vi "FetchMultiPoint.vi"(8 "error in (no error)":errorcluster, 11 "NISTSimulation in":refnum<class "Simulation.lvclass">) -> (0 "error out":errorcluster, 3 "NISTSimulation out":refnum<class "Simulation.lvclass">)   [LabVIEW 2014, in "SamplerPlugins.lvlib" / "Simulation.lvclass"]
uses:
  Simulation.lvclass
  NISTSamplerPluginsBaseClass/TypeDefs/MultiPointReadingParams.ctl
  NISTSamplerPluginsBaseClass/SamplerPluginsBase.lvclass
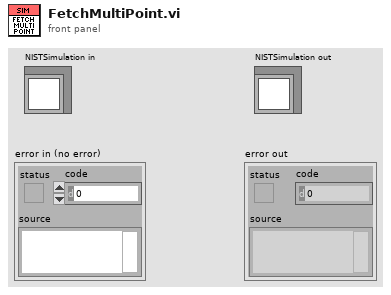
[diagram p1: front panel]
types:
  T1 = typedef "SamplerPlugins.lvlib/SamplerPluginsBase.lvclass/ReadMultiPointParams.ctl" = cluster{"iMaxTimeMilliseconds":i32, "iArraySize":i32}
  T2 = typedef "SamplerPlugins.lvlib/SamplerPluginsBase.lvclass/ConfigMultiPointParams.ctl" = cluster{"iTriggerCount":i32, "iSampleCount":i32, "eSampleClock":u16, "dSampleInterval":dbl}
  T3 = typedef "SamplerPlugins.lvlib/SamplerPluginsBase.lvclass/MultiPointReadingParams.ctl" = cluster{"dReadingArray":dbl[], "iActualPts":i32, "Timestamp":dbl}
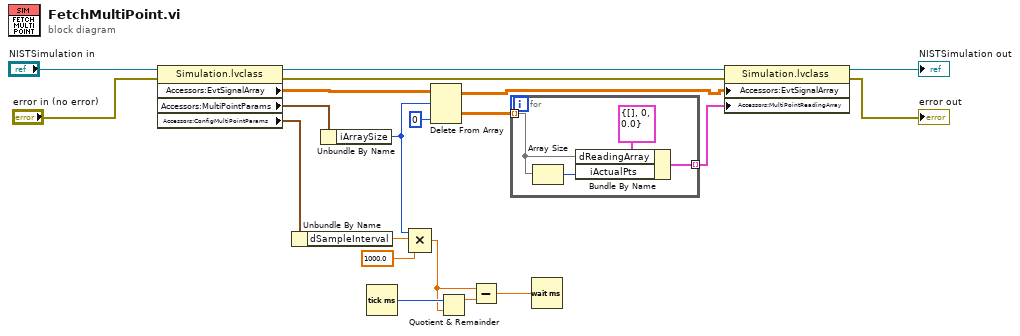
[diagram p0: block diagram]
diagram:
  n1 = property class="Simulation.lvclass"(reference="NISTSimulation in", error in="error in (no error)") -> (reference out=w15:refnum<class "Simulation.lvclass">, error out=w10:errorcluster, "Accessors:EvtSignalArray"=w17:dbl[][], "Accessors:MultiPointParams"=w18:T1, "Accessors:ConfigMultiPointParams"=w9:T2)
  n2 = Unbundle By Name(w9) -> ("dSampleInterval"=w8:dbl)
  n3 = Unbundle By Name(w18) -> ("iArraySize"=w6:i32)
  n4 = Tick Count (ms)() -> (millisecond timer value=w4:u32)
  n5 = Compound Arithmetic op=MULTIPLY(w6, w8, 1000.0 ("y")) -> (w2:dbl)
  n6 = Delete From Array(array=w17, length=w6, index (col)=0 ("disabled index (col)")) -> (deleted portion=w5:dbl[][], array with subset deleted=w14:dbl[][])  [unwired: 1 in]
  n7 = Quotient & Remainder(x=w4, y=w2) -> (x-y*floor(x/y)=w3:dbl)  [unwired: 1 out]
  n8 = Subtract(x=w2, y=w3) -> (x-y=w1:dbl)
  n9 = for {
    tunnel: w5 -> [w22] mode=indexing
    tunnel: [w21] -> w13 mode=indexing
    n10 = Array Size(array=w22) -> (size(s)=w23:i32)
    n11 = Bundle By Name(cluster=T3 {"dReadingArray"=[], "iActualPts"=0, "Timestamp"=0.0} ("MultiPointReadingParams"), "dReadingArray"=w22, "iActualPts"=w23) -> (w21:T3)
  }
  n12 = Wait (ms)(milliseconds to wait=w1) -> ()  [unwired: 1 out]
  n13 = property class="Simulation.lvclass"(reference=w15, error in=w10, "Accessors:EvtSignalArray"=w14, "Accessors:MultiPointReadingArray"=w13) -> (reference out=→"NISTSimulation out":refnum<class "Simulation.lvclass">, error out=→"error out":errorcluster)
